vi "Get Type.vi"(8 "error in (no error)":errorcluster, 11 "Source Instr in":refnum<class "Source Instr.lvclass">) -> (0 "error out":errorcluster, 2 "Type":string, 3 "Source Instr out":refnum<class "Source Instr.lvclass">)   [LabVIEW 2015, in "Item Actor.lvlib" / "Source Instr.lvclass"]
uses:
  Source Instr.lvclass
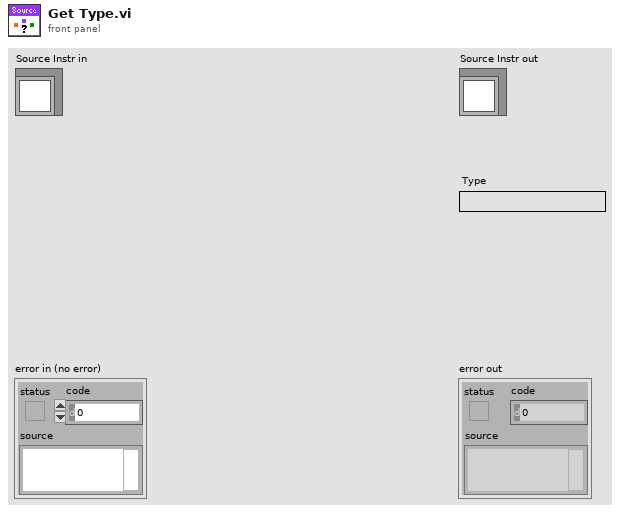
[diagram p1: front panel]
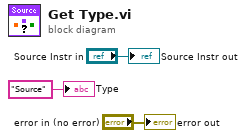
[diagram p0: block diagram]
diagram:
  "error out" <- "error in (no error)"
  "Source Instr out" <- "Source Instr in"
  "Type" <- "Source" ("Type")
